vi "read1Byte Rx.vi"(10 "protocol_version":i32, 11 "port_num":i32) -> (3 "function return":u8)   [LabVIEW 2015, in "dxl_x86_c.lvlib"]
doc: "WINDECLSPEC uint8_t read1ByteRx (int port_num, int protocol_version);"
uses:
  dxl_x86_c.lvlib
  dxl_x86_c.dll
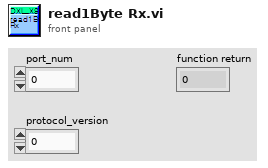
[diagram p1: front panel]
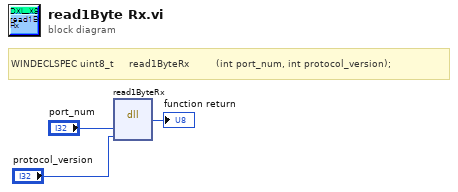
[diagram p0: block diagram]
diagram:
  # "WINDECLSPEC uint8_t     read1ByteRx         (int port_num, int protocol_version);"
  n1 = dll-call lib="C:/Users/Platform/Desktop/LabVIEW/dxl_x86_c.lvlib/dxl_x86_c.*" fn="read1ByteRx"("port_num"="port_num", "protocol_version"="protocol_version") -> (→"function return":u8)  [unwired: 5 in, 2 out]
